vi "Recall AP Sx Panel.vi"(8 "error in (no error)":errorcluster caption="错误输入（无错误）", 9 "restoreWindows":i32, 10 "asicName":string, 11 "asicHandle":i32) -> (0 "error out":errorcluster caption="错误输出", 2 "asicName out":string, 3 "function return":i32)   [LabVIEW 2018]
doc: "extern int __stdcall RecallAPSxPanel (int asicHandle, IN char * asicName, IN BOOL restoreWindows);"
uses:
  APSx.dll/APSx.dll
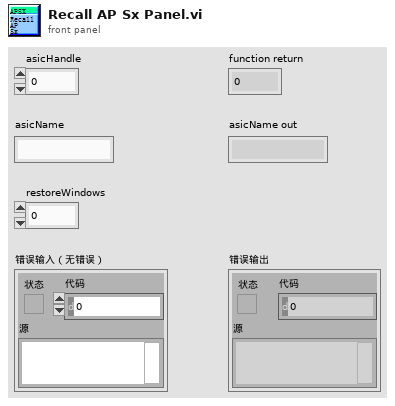
[diagram p1: front panel]
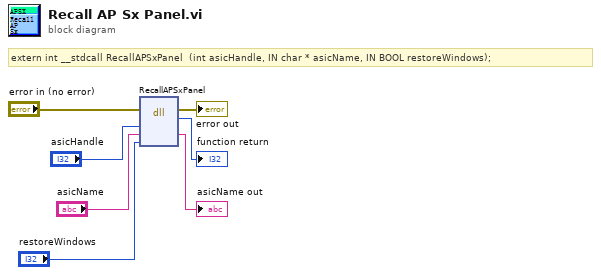
[diagram p0: block diagram]
diagram:
  # "extern int __stdcall RecallAPSxPanel  (int asicHandle, IN char * asicName, IN BOOL restoreWindows);"
  n1 = dll-call lib="PTH2[abs D项目Feng恒隆项目Labview传感器对中台SourcesAPSx.dllAPSx.*" fn="RecallAPSxPanel"(error in="error in (no error)", "asicHandle"="asicHandle", "asicName"="asicName", "restoreWindows"="restoreWindows") -> (error out=→"error out":errorcluster, →"function return":i32, "asicName"=→"asicName out":string)  [unwired: 4 in, 1 out]
